vi "OAT Polar Set Default Cursor Positions.vi"(6 "cursor attributes":T2={"layout color"=852223, "active color"=16740820, "precision"=2, "BG transparent? (T)"=FALSE, "radius"=2}, 7 "polar attributes":T1={"maximum"=1.0, "minimum"=0.0, "clip to min"=FALSE, "log"=FALSE, "grid color"=0, "plot color"=0, "fmt and prec"={"format"=enum."Decimal", "precision"=2}, "visible section"=8} {"minimum" format="%.2f"; "maximum" format="%.4f"}, 8 "Max number of labels\nalong radius":i32=5, 9 "cursor values":dbl[](array[numeric]) format="%.2f", 10 "phases":dbl[](array[numeric]) format="%.2f", 11 "magnitudes (even angular)":dbl[](array[numeric]) format="%.2f") -> (3 "Cursor List (EU position]":T3(array[cluster]) {"Location"."phase" format="%.2f"; "Location"."mag" format="%.2f"})   [LabVIEW 2017]
uses:
  <vilib>/addons/Sound and Vibration/Order Analysis/Backward Compatibility/SubVIs/OAT Polar Cursor Attributes.ctl
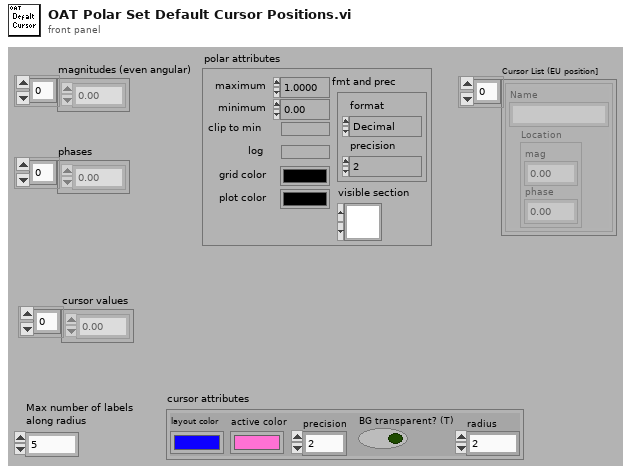
[diagram p1: front panel]
types:
  T1 = cluster{"maximum":dbl, "minimum":dbl, "clip to min":bool, "log":bool, "grid color":u32, "plot color":u32, "fmt and prec":cluster{"format":enum8{"Decimal", "Scientific", "Engineering", "Binary", "Octal", "Hex"}, "precision":u8}, "visible section":u16}
  T2 = typedef "OAT Polar Cursor Attributes.ctl" = cluster{"layout color":u32, "active color":u32, "precision":i16, "BG transparent? (T)":bool, "radius":i16}
  T3 = cluster{"Name":string, "Location":cluster{"mag":dbl, "phase":dbl}}[]
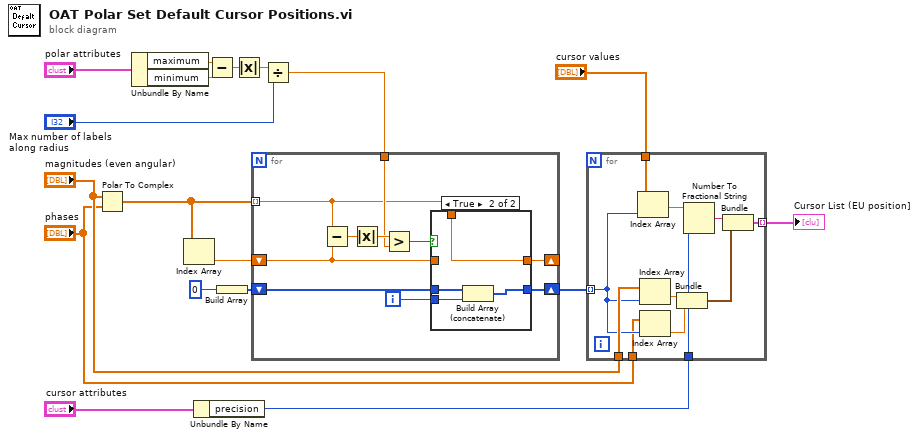
[diagram p0: block diagram]
diagram:
  n1 = Polar To Complex(1:"phases", 2:"magnitudes (even angular)") -> (0:w6:cdb[])
  n2 = Unbundle By Name("polar attributes") -> ("maximum"=w16:dbl, "minimum"=w15:dbl)
  n3 = Index Array(array=w6) -> (element=w5:cdb)  [unwired: 1 in]
  n4 = Unbundle By Name("cursor attributes") -> ("precision"=w11:i16)
  n5 = Subtract(x=w16, y=w15) -> (x-y=w14:dbl)
  n6 = Build Array(0 ("element")) -> (w8:i32[])
  n7 = Absolute Value(x=w14) -> (abs(x)=w13:dbl)
  n8 = Divide(x=w13, y="Max number of labels\nalong radius") -> (x/y=w7:dbl)
  n9 = for {
    tunnel: w7 -> [w26]
    shift-right: [w23] -> w9
    shift-left: w8 -> [w24]
    tunnel: w6 -> [w22] mode=indexing
    shift-right: [w21] -> _
    shift-left: w5 -> [w20]
    i -> [w19]
    n10 = Subtract(x=w22, y=w20) -> (x-y=w28:cdb)
    n11 = Absolute Value(x=w28) -> (abs(x)=w27:dbl)
    n12 = Greater?(x=w27, y=w26) -> (0:w25:bool)
    n13 = case shown="True" w25 {
      tunnel: w24 -> [w30 w34]
      tunnel: w22 -> [_ w31]
      tunnel: [w30 w33] -> w23
      tunnel: [w29 w31] -> w21
      tunnel: w20 -> [w29 _]
      tunnel: w19 -> [_ w32]
      frame False {
      }
      frame True {
        n14 = Build Array (concatenate)(w34, w32) -> (w33:i32[])
      }
    }
  }
  n15 = for {
    tunnel: w11 -> [w45]
    tunnel: w9 -> [w38] mode=indexing
    tunnel: [w42] -> w10 mode=indexing
    tunnel: "cursor values" -> [w40]
    tunnel: "magnitudes (even angular)" -> [w39]
    tunnel: "phases" -> [w37]
    n16 = Index Array(array=w40, index=w38) -> (element=w41:dbl)
    n17 = Index Array(array=w39, index=w38) -> (element=w36:dbl)
    n18 = Index Array(array=w37, index=w38) -> (element=w35:dbl)
    n19 = Bundle(w36, w35) -> (w43:cluster{dbl, dbl})  [unwired: 1 in]
    n20 = Number To Fractional String(number=w41, precision (6)=w45) -> (F-format string=w44:string)  [unwired: 2 in]
    n21 = Bundle(w44, w43) -> (w42:cluster{string, cluster{dbl, dbl}})  [unwired: 1 in]
  }
  "Cursor List (EU position]" <- w10
